vi "Fetch Single Record Binary.vi"(0 "device session in":refnum<class "Device Session.lvclass">, 1 "starting record":u64, 5 "fetch relative to":T3=enum."First Pretrigger Sample", 7 "number of samples":u64=1000, 9 "timeout (ms)":i32=1000, 11 "error in":errorcluster, 12 "fetch offset":i64) -> (4 "device session out":refnum<class "Device Session.lvclass">, 6 "data":i16[][](array[numeric]), 8 "relativeX (samples)":dbl, 10 "scaling coefficients":T1[](array[typedef]), 14 "requested record info":T2={"number of samples"=0, "starting sample number"=0, "number of channels"=1, "timestamps"=[]}, 15 "error out":errorcluster)   [LabVIEW 2021, in "Device Session.lvclass"]
doc: "Fetches binary data from a single record in an acquisition. No data is returned if this VI times out. You must run the <B>Initiate</B> VI before running this VI.\n\n<B>Input Parameters</B>\n\n<B>device session in</B> is a reference to the Device Session object, which contains a session to each instrument design library used in this sample project. This parameter is obtained from the 'Open Session' VI.\n\n<B>starting record</B> specifies the record to retrieve. Index of the record numbers starts at 0.\n\n<B>fetch relative to</B> specifies the relative location within the acquired record from where the VI begins to fetch data.\n\n'First Sample': the fetch starts at the first sample acquired by the device. If the device wraps data in its memory buffer, the first sample is no longer available. In this case, the VI returns an error if 'fetch offset' specifies a location that is within the overwritten portion of the memory buffer.\n'Reference Trigger Sample': the fetch starts relative to the Reference Trigger.\n'First Pretrigger Sample': the fetch starts relative to the first pretrigger sample acquired. If you do not configure a Reference Trigger, 'First Pretrigger Sample' behaves the same as 'First Sample' because there are no pretrigger samples.\n'Most Recent Sample': the fetch starts relative to the most recently acquired sample. The value of 'fetch offset' must be negative. This VI doesn't support this option. Consider using the 'Fetch Single Record' VI instead.\n'Current Read Position': the fetch starts after the last fetched sample. This VI doesn't support this option. Consider using the 'Fetch Single Record' VI instead.\n\n<B>number of samples</B> specifies the number of samples to fetch. The default value is 1000.\n\n<B>timeout (ms)</B> specifies the time, in milliseconds, allotted for the Fetch Multiple Records VI to complete execution of each record before returning a timeout error. A value of -1 specifies that the VI waits until all data is available. A value of 0 is not supported. The default value is 10,000. You cannot abort a pending fetch using the Abort VI or Close VI.\n\n<B>fetch offset</B> specifies the offset relative to the position, which is specified by the 'fetch relative to' parameter, from which to start fetching data. Offset can be a positive or negative value. The default value is 0.\n\n<B>error in</B> describes error conditions that occur before this node runs. This input provides standard 'error in' functionality.\n\n<B>Output Parameters</B>\n\n<B>device session out</B> passes a reference to the session to the next VI.\n\n<B>data</B> returns the fetched binary data.\n\n<B>requested record info</B> returns the record parameters configuration.\n\n<B>scaling coefficients</B> returns the scaling coefficients for the channels selected for acquisition.\n\n<B>relativeX (samples)</B> returns the relative position from the trigger to the first sample in the acquired data.\n\n<B>error out</B> contains error information. This output provides standard 'error out' functionality."
uses:
  Device Session.lvclass
  <instrlib>/_niInstr/Multirecord Acquisition/Interface/v1/Host/Public/Fetch Relative To Enum.ctl
  <instrlib>/_niInstr/Multirecord Acquisition/Interface/v1/Host/Public/Requested Record Info.ctl
  <instrlib>/_niInstr/Multirecord Acquisition/Interface/v1/Host/Public/Scaling Coefficient.ctl
  Device Session.lvclass/Device Session.ctl
  <instrlib>/_niInstr/Multirecord Acquisition/Interface/v1/Host/Private/Fetch Single Record I16 NCh Wrapper.vi
  <instrlib>/HSAI-RIO/Config/Group A/v1/Host/Main/niHSAI Group A Config v1 Host.lvclass
  <instrlib>/_niInstr/Multirecord Acquisition/Interface/v1/Host/niInstr Multirecord Acquisition v1 Host.lvclass
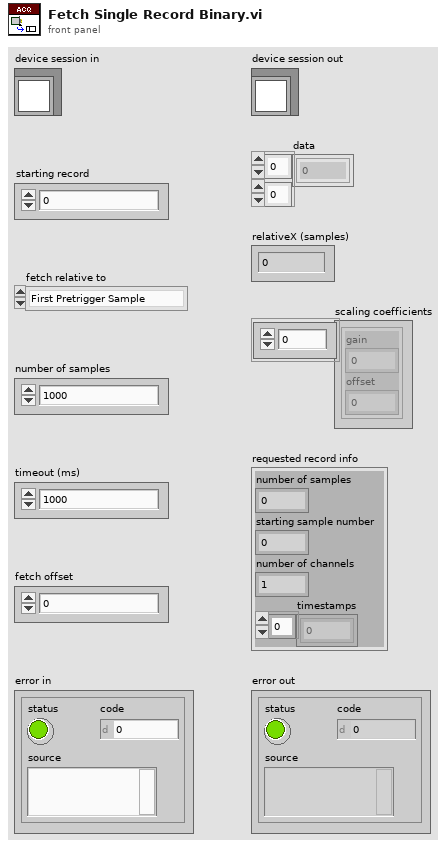
[diagram p1: front panel]
types:
  T1 = typedef "niInstr Multirecord Acquisition v1 Host.lvclass/Scaling Coefficient.ctl" = cluster{"gain":dbl, "offset":dbl}
  T2 = typedef "niInstr Multirecord Acquisition v1 Host.lvclass/Requested Record Info.ctl" = cluster{"number of samples":u64, "starting sample number":u64, "number of channels":u64, "timestamps":u64[]}
  T3 = typedef "niInstr Multirecord Acquisition v1 Host.lvclass/Fetch Relative To Enum.ctl" = enum16{"First Sample", "Reference Trigger Sample", "First Pretrigger Sample", "Most Recent Sample", "Current Read Position"}
  T4 = typedef "Device Session.lvclass/Device Session Object.ctl" = cluster{"fpga reference":T5, "reg bus":refnum<class "niInstr FIFO Register Bus v1 Host.lvclass">, "subsystem map":refnum<class "niInstr Subsystem Map v1 Host.lvclass">, "cal data":refnum<class "niHSAI Cal Data v1 Host.lvclass">, "config":refnum<class "niHSAI Group A Config v1 Host.lvclass">, "acquisition 0":refnum<class "niInstr Multirecord Acquisition v1 Host.lvclass">, "acquisition 1":refnum<class "niInstr Multirecord Acquisition v1 Host.lvclass">, "number of selected acq channels":u8, "selected acq channels":bool[], "number of channels":u32, "configured channels":bool[], "acq configuration":cluster{"number of samples":u64, "number of records":u64, "pretrigger samples":u64}, "actual channel configuration":T6[], "sample clock rate (Hz)":dbl, "scaling coefficients":T1[]}
  T5 = typedef "Device Session.lvclass/FPGA Refnum.ctl" = refnum<k20>
  T6 = typedef "niHSAI Types v1 Host.lvlib/Channel Configuration.ctl" = cluster{"channel":u32, "coupling":T7, "impedance":T8, "bandwidth":T9, "vertical range":dbl, "vertical offset":dbl}
  T7 = typedef "niHSAI Types v1 Host.lvlib/Coupling.ctl" = enum8{"Default", "DC", "AC"}
  T8 = typedef "niHSAI Types v1 Host.lvlib/Impedance.ctl" = enum8{"Default", "1 mega ohm", "50 ohm"}
  T9 = typedef "niHSAI Types v1 Host.lvlib/Bandwidth.ctl" = enum8{"Default", "Full Bandwidth", "Anti-alias Filter", "150 MHz"}
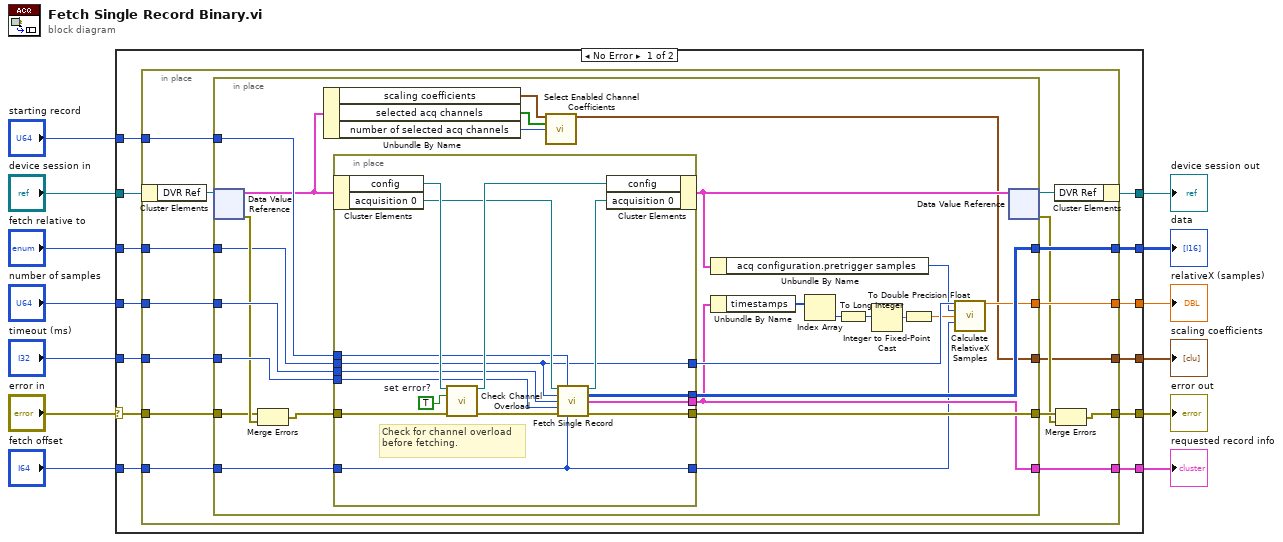
[diagram p0: block diagram]
diagram:
  n1 = case shown="No Error" "error in" {
    selector: "error in" -> [w26 w84]
    tunnel: [w21 w84] -> w3
    tunnel: "device session in" -> [w16 w83]
    tunnel: [w15 w83] -> w6
    tunnel: "number of samples" -> [w25 _]
    tunnel: "timeout (ms)" -> [w24 _]
    tunnel: "fetch offset" -> [w23 _]
    tunnel: "starting record" -> [w22 _]
    tunnel: "fetch relative to" -> [w20 _]
    tunnel: [w19 _] -> w5
    tunnel: [w18 _] -> w4
    tunnel: [w17 _] -> w2
    tunnel: [w14 _] -> w1
    frame No Error {
      n2 = in-place {
        in-place-border: w26 -> [w41]
        in-place-border: w25 -> [w40]
        in-place-border: w24 -> [w39]
        in-place-border: w23 -> [w38]
        in-place-border: w22 -> [w37]
        in-place-border: [w36] -> w21
        in-place-border: w20 -> [w34]
        in-place-border: [w33] -> w19
        in-place-border: [w32] -> w18
        in-place-border: [w31] -> w17
        in-place-border: [w27] -> w14
        n3 = in-place-cluster #1(w16) -> ("DVR Ref"=w29:refnum<data-value>)
        n4 = in-place {
          in-place-border: w41 -> [w63]
          in-place-border: [w67] -> w35
          in-place-border: w40 -> [w66]
          in-place-border: w39 -> [w65]
          in-place-border: w38 -> [w51]
          in-place-border: w37 -> [w60]
          in-place-border: w34 -> [w49]
          in-place-border: [w59] -> w33
          in-place-border: [w58] -> w32
          in-place-border: [w47] -> w31
          in-place-border: [w42] -> w27
          n5 = in-place-dvr #2(w29) -> (w50:T4, w64:errorcluster)
          n6 = Merge Errors(w63, w64) -> (w52:errorcluster)
          n7 = Unbundle By Name(w50) -> ("scaling coefficients"=w57:T1[], "selected acq channels"=w62:bool[], "number of selected acq channels"=w61:u8)
          n8 = in-place {
            in-place-border: [w82] -> w67
            in-place-border: w66 -> [w71]
            in-place-border: w65 -> [w70]
            in-place-border: w60 -> [w72]
            in-place-border: [w79] -> w59
            in-place-border: [w78] -> w47
            in-place-border: w52 -> [w77]
            in-place-border: w49 -> [w69]
            in-place-border: w51 -> [w68]
            in-place-border: [w69] -> w48
            in-place-border: [w68] -> w46
            w80 = TRUE  # set error?
            # "Check for channel overload before fetching."
            n9 = in-place-cluster #3(w50) -> ("config"=w76:refnum<class "niHSAI Group A Config v1 Host.lvclass">, "acquisition 0"=w74:refnum<class "niInstr Multirecord Acquisition v1 Host.lvclass">)
            n10 = call-dynamic "Check Channel Overload.vi"("session in"=w76, "set error? (T)"=w80, "error in"=w77) -> ("session out"=w75:refnum<class "niHSAI Group A Config v1 Host.lvclass">, "error out"=w81:errorcluster)  [unwired: 10 in, 1 out]
            n11 = call-poly <instrlib>:"Fetch Single Record.vi"("session in"=w74, "record number"=w72, "fetch relative to"=w69, "number of samples"=w71, "timeout (ms)"=w70, "error in"=w81, "fetch offset"=w68) -> ("session out"=w73:refnum<class "niInstr Multirecord Acquisition v1 Host.lvclass">, "data"=w79:i16[][], "requested record info"=w78:T2, "error out"=w82:errorcluster)  [unwired: 5 in]
            n12 = in-place-cluster #3("config"=w75, "acquisition 0"=w73) -> (w44:T4)
          }
          n13 = call "Select Enabled Channel Coefficients.vi"("configured scaling coefficients"=w57, "selected acq channels to store"=w62, "number of selected acq channels to store"=w61) -> ("stored scaling coefficients"=w42:T1[])  [unwired: 12 in]
          n14 = Unbundle By Name(w44) -> ("acq configuration.pretrigger samples"=w43:u64)
          n15 = Unbundle By Name(w47) -> ("timestamps"=w54:u64[])
          n16 = Index Array(array=w54) -> (element=w53:u64)  [unwired: 1 in]
          n17 = To Long Integer(number=w53) -> (32bit integer=w55:i32)
          n18 = Integer to Fixed-Point Cast(integer=w55) -> (fixed-point=w56:fxp<+/-,32,5>)  [unwired: 1 in]
          n19 = To Double Precision Float(number=w56) -> (double precision float=w45:dbl)
          n20 = call "Calculate RelativeX Samples.vi"("fetch relative to"=w48, "pretrigger samples"=w43, "timestamps"=w45, "fetch offset"=w46) -> ("relativeX (samples)"=w58:dbl)  [unwired: 11 in]
          n21 = in-place-dvr #2(w44) -> (w28:refnum<data-value>, w30:errorcluster)
        }
        n22 = in-place-cluster #1("DVR Ref"=w28) -> (w15:refnum<class "Device Session.lvclass">)
        n23 = Merge Errors(w35, w30) -> (w36:errorcluster)
      }
    }
    frame Error {
    }
  }
  "error out" <- w3
  "device session out" <- w6
  "data" <- w5
  "requested record info" <- w2
  "relativeX (samples)" <- w4
  "scaling coefficients" <- w1
